vi "Player Increment Score.vi"(8 "error in (no error)":errorcluster, 10 "Amount":u32, 11 "Player in":refnum<class "Player.lvclass">) -> (0 "error out":errorcluster, 3 "Player out":refnum<class "Player.lvclass">)   [LabVIEW 2019, in "Player.lvclass"]
uses:
  Player.lvclass
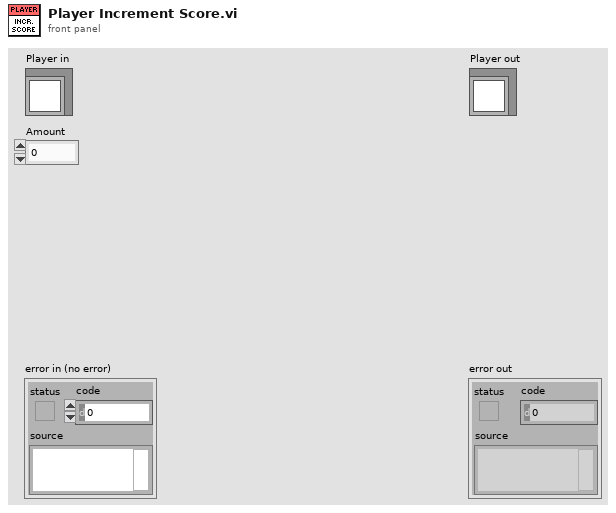
[diagram p1: front panel]
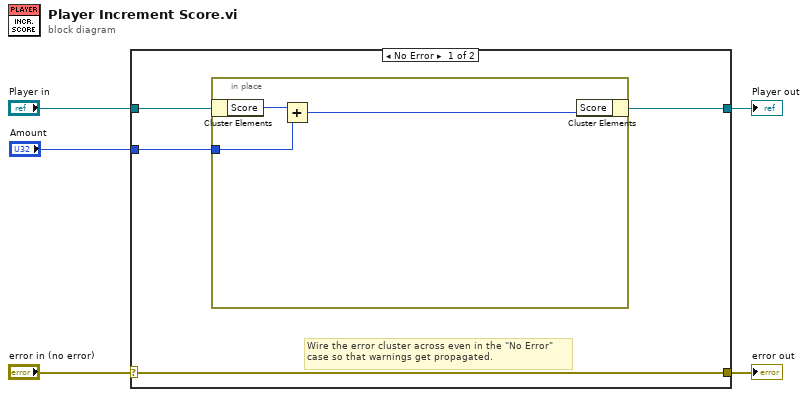
[diagram p0: block diagram]
diagram:
  n1 = case shown="No Error" "error in (no error)" {
    selector: "error in (no error)" -> [w9 w14]
    tunnel: [w9 w14] -> w4
    tunnel: [w8 w13] -> w2
    tunnel: "Player in" -> [w7 w13]
    tunnel: "Amount" -> [w6 _]
    frame No Error {
      # "Wire the error cluster across even in the \"No Error\"\ncase so that warnings get propagated."
      n2 = in-place {
        in-place-border: w6 -> [w11]
        n3 = in-place-cluster #1(w7) -> ("Score"=w12:u32)
        n4 = Add(x=w12, y=w11) -> (x+y=w10:u32)
        n5 = in-place-cluster #1("Score"=w10) -> (w8:refnum<class "Player.lvclass">)
      }
    }
    frame Error {
    }
  }
  "error out" <- w4
  "Player out" <- w2
